vi "Simple Reader.vi"(8 "error in (no error)":errorcluster, 11 "temperature reader in":refnum<class "temperature reader.lvclass">) -> (0 "error out":errorcluster, 2 "Signals":dbl[](array[numeric]), 3 "temperature reader out":refnum<class "temperature reader.lvclass">)   [LabVIEW 2018, in "temperature reader.lvclass"]
uses:
  temperature reader.lvclass
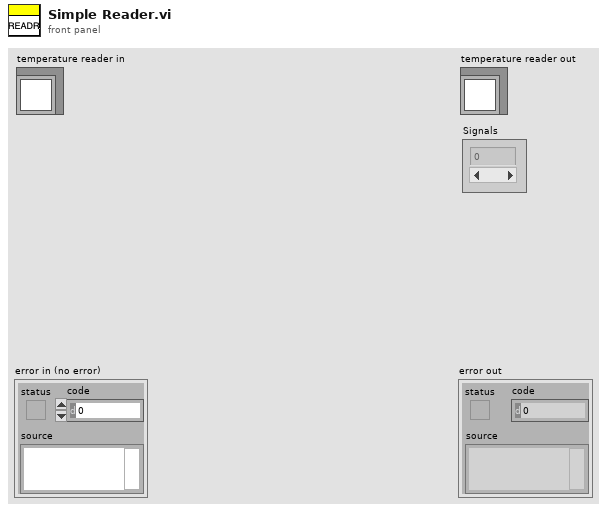
[diagram p1: front panel]
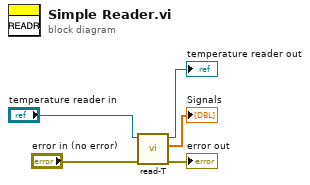
[diagram p0: block diagram]
diagram:
  n1 = call "read-T.vi"("error in (no error)"="error in (no error)", "temperature reader.lvclass"="temperature reader in") -> ("error out"=→"error out":errorcluster, "Result"=→"Signals":dbl[], "temperature reader.lvclass Out"=→"temperature reader out":refnum<class "temperature reader.lvclass">)  [unwired: 7 in]
